vi "Get Control Information.vi"(8 "error in (no error)":errorcluster, 11 "String in":refnum<class "String.lvclass">) -> (0 "error out":errorcluster, 2 "Control Information":string[][](array[string]), 3 "String out":refnum<class "String.lvclass">)   [LabVIEW 2017, in "Localization.lvlib" / "String.lvclass"]
doc: "VI for override that is supposed to do go throgh the process for each control type and pull out the information that is necessary for each control.\n\nChoose Movement Consulting, LLC"
uses:
  String.lvclass
  C:/Apps/CMC/OpenSource/Localization/Control Info/Control Info.lvclass
  Localization.lvlib
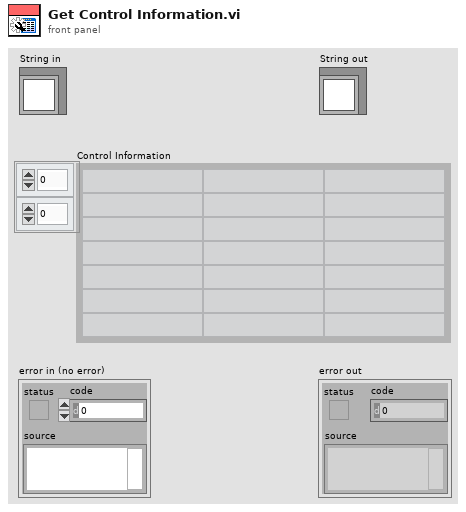
[diagram p1: front panel]
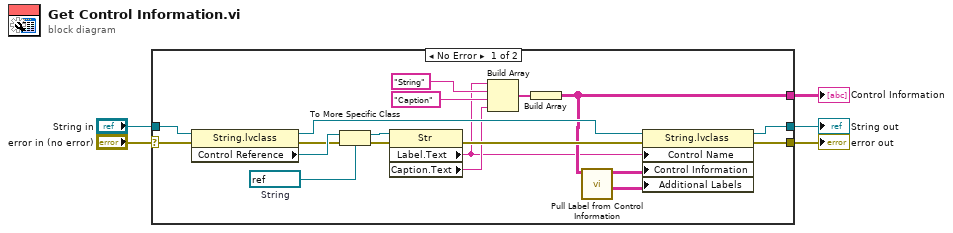
[diagram p0: block diagram]
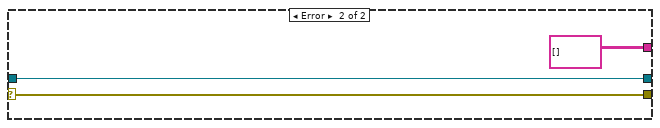
[diagram p2: hidden frame]
diagram:
  n1 = case shown="No Error" "error in (no error)" {
    selector: "error in (no error)" -> [w15 w26]
    tunnel: "String in" -> [w18 w27]
    tunnel: [w9 string[][] []] -> w3
    tunnel: [w13 w26] -> w2
    tunnel: [w12 w27] -> w1
    frame No Error {
      w24 = refnum<vi> refnum  # String
      n2 = property class="String.lvclass"(reference=w18, error in=w15) -> (reference out=w14:refnum<class "String.lvclass">, error out=w16:errorcluster, "Control Reference"=w17:refnum<vi>)
      n3 = To More Specific Class(target class=w24, reference=w17, error in=w16) -> (specific class reference=w23:refnum<vi>, error out=w19:errorcluster)
      n4 = property class="Str"(reference=w23, error in=w19) -> (error out=w11:errorcluster, "Label.Text"=w7:string, "Caption.Text"=w10:string)  [unwired: 1 out]
      n5 = Build Array(w7, "String", "Caption", w10) -> (w20:string[])
      n6 = Build Array(w20) -> (w9:string[][])
      n7 = call "Pull Label from Control Information.vi"("Control Caption Table"=w9) -> ("Additional Labels"=w6:string[][], "Control Information"=w8:string[][])  [unwired: 9 in]
      n8 = property class="String.lvclass"(reference=w14, error in=w11, "Control Name"=w7, "Control Information"=w8, "Additional Labels"=w6) -> (reference out=w12:refnum<class "String.lvclass">, error out=w13:errorcluster)
    }
    frame Error {
    }
  }
  "error out" <- w2
  "String out" <- w1
  "Control Information" <- w3
